vi "Configurator.vi"(8 "error in (no error)":errorcluster) -> (0 "error out":errorcluster)   [LabVIEW 2014]
uses:
  <vilib>/userdefined/High Color/IMAQdx.ctl
  ImageCluster.ctl
  <vilib>/vision/Image Controls.llb/IMAQ Image.ctl
  STD - Tap Mode.ctl
  FlappyHeightPoint.ctl
  <vilib>/LabVIEW Hacker/LINX/Private/Type Defs/User Platform.ctl
  <vilib>/LabVIEW Hacker/LINX/Private/Type Defs/Interface.ctl
  <vilib>/vision/driver/IMAQdx.llb/IMAQdx Acquisition Mode.ctl
  Globals.vi
  <vilib>/vision/driver/NI_Vision_Acquisition_Software.lvlib
  <vilib>/LabVIEW Hacker/LINX/LVH-LINX.lvlib
panel:
  in  "Proceed":bool
  out "Camera connected":bool
  out "Arduino connected":bool
  out "Flappy template loaded":bool
  out "Pipe template loaded":bool
  in  "Serial Port":refnum<visa-resource-name>="N/A"
  in  "IMAQdx Camera Session":T1 caption="Camera to use"
  out "Camera Information Array":T2(array[cluster]) {"BusType" format="%x"; "SerialNumberLow" format="%.0x"; "SerialNumberHigh" format="%.0x"}
  in  "Pipe Corner Template Path":path
  in  "Flappy Template Path":path
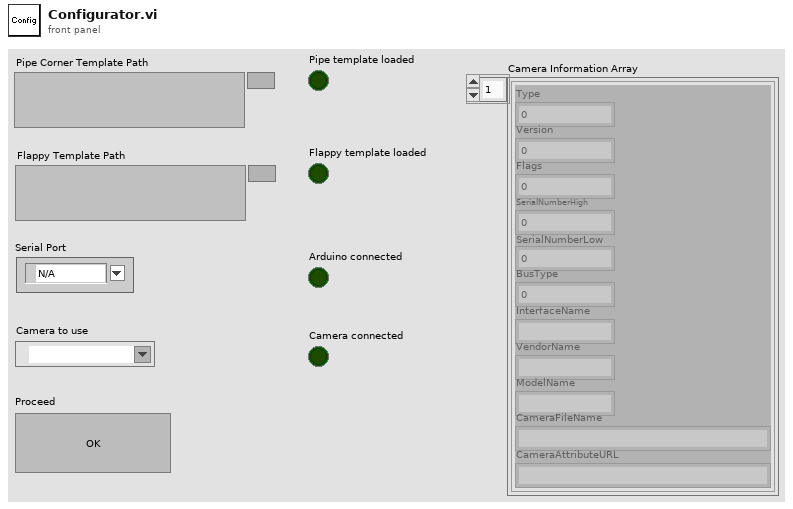
[diagram p1: front panel]
types:
  T1 = typedef "IMAQdx.ctl" = refnum<k21>
  T2 = cluster{"Type":u32, "Version":u32, "Flags":u32, "SerialNumberHigh":u32, "SerialNumberLow":u32, "BusType":u32, "InterfaceName":string, "VendorName":string, "ModelName":string, "CameraFileName":string, "CameraAttributeURL":string}[]
  T3 = typedef "FlappyHeightPoint.ctl" = cluster{"Time (s)":dbl, "Height (px)":dbl}
  T4 = typedef "STD - Tap Mode.ctl" = enum32{"No Action", "Stay Level", "Rise", "Fall", "Calibrate"}
  T5 = typedef "ImageCluster.ctl" = cluster{"Screenshot":T6, "Time (s)":dbl}
  T6 = typedef "IMAQ Image.ctl" = refnum<image>
  T7 = typedef "LVH-LINX.lvlib/Interface.ctl" = enum16{"Serial", "TCP"}
  T8 = typedef "LVH-LINX.lvlib/User Platform.ctl" = enum16{"Default", "LINX", "myRIO"}
  T9 = typedef "NI_Vision_Acquisition_Software.lvlib/IMAQdx Acquisition Mode.ctl" = enum32{"One Shot", "Continuous"}
  T10 = typedef "LVH-LINX.lvlib/LINX Ref.ctl" = cluster{"Platform":T11, "Interface":T7, "LINX Device Config":T12}
  T11 = typedef "LVH-LINX.lvlib/Platform.ctl" = enum16{"LINX", "myRIO"}
  T12 = typedef "LVH-LINX.lvlib/Device.lvlib/LINX Device Config.ctl" = cluster{"Interface":T7, "COM Port":refnum<visa-resource-name>, "TCP Configuration":T13, "Device Family":T14, "Device ID":u8, "Device Name":string, "TCP Ref":refnum<k5>}
  T13 = typedef "LVH-LINX.lvlib/Device.lvlib/TCP Config.ctl" = cluster{"IP Address":string, "Port":u16}
  T14 = typedef "LVH-LINX.lvlib/Device Family.ctl" = enum8{"National Instruments", "Digilent", "Arduino"}
  T15 = typedef "Image Type" = u32
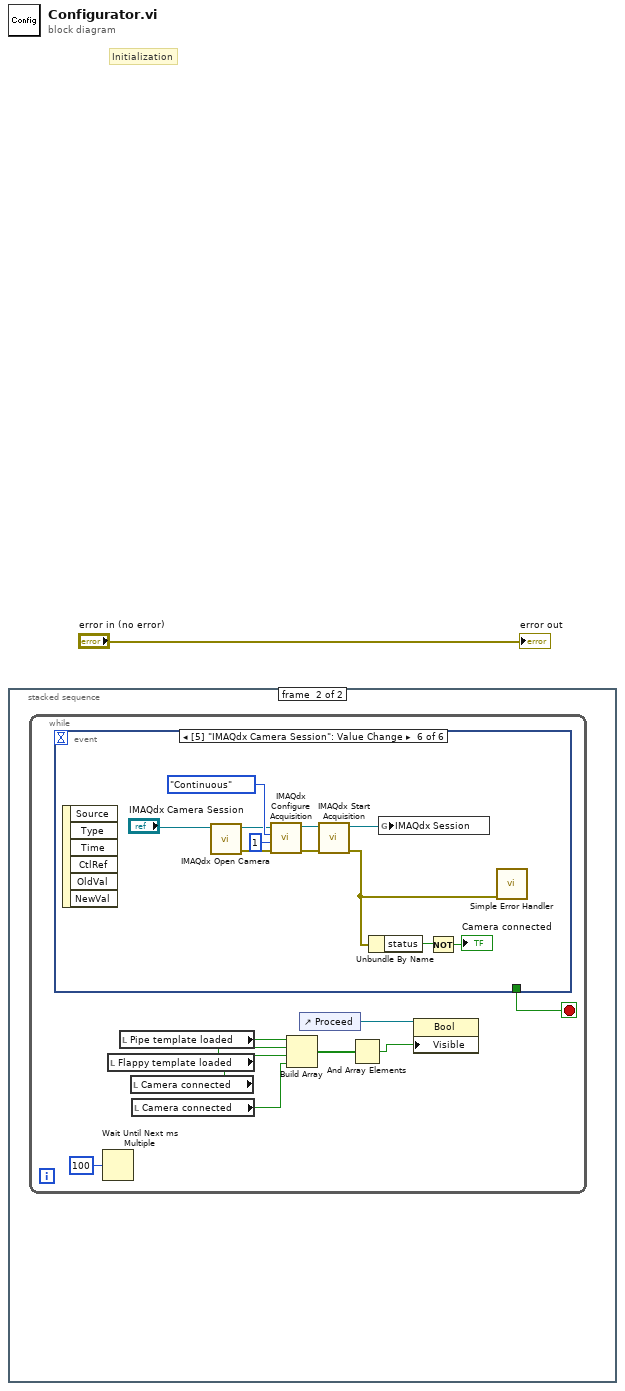
[diagram p0: block diagram]
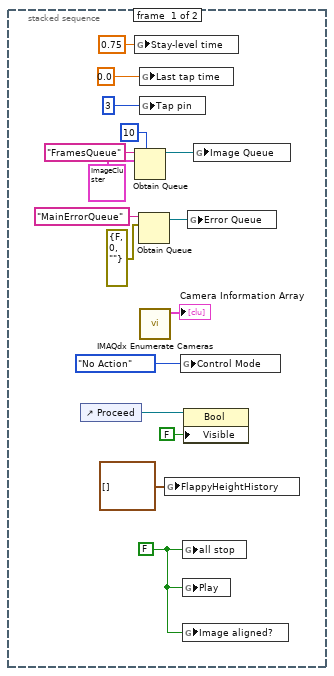
[diagram p2: hidden frame]
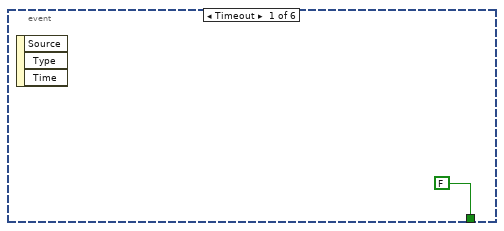
[diagram p3: hidden frame]
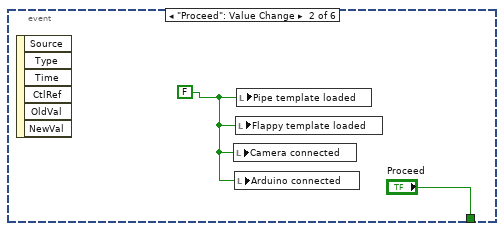
[diagram p4: hidden frame]
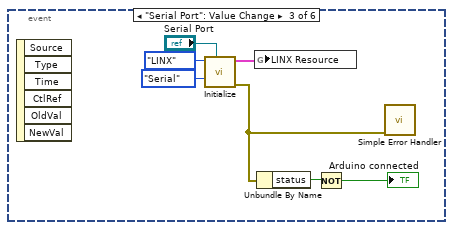
[diagram p5: hidden frame]
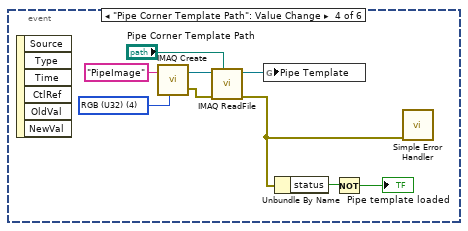
[diagram p6: hidden frame]
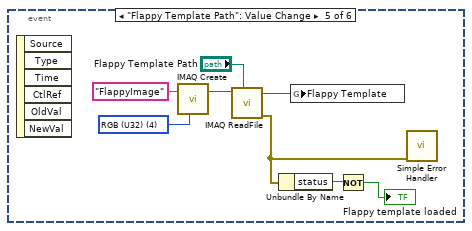
[diagram p7: hidden frame]
diagram:
  # "Initialization"
  n1 = stacked-sequence {
    frame #0 {
      w2 = FALSE ("all stop")
      n2 = control-ref of="Proceed"() -> (w5:refnum<vi>)
      n3 = global write "Globals.vi" "Stay-level time"(0.75 ("Stay-level time")) -> ()
      n4 = Obtain Queue(max queue size (-1, unlimited)=10, name (unnamed)="FramesQueue", element data type=T5 {"Screenshot"=refnum, "Time (s)"=0.0}) -> (queue out=w14:refnum<queue>)  [unwired: 2 in, 2 out]
      n5 = Obtain Queue(name (unnamed)="MainErrorQueue", element data type=errorcluster {"status"=FALSE, "code"=0, "source"=""} ("error constant")) -> (queue out=w8:refnum<queue>)  [unwired: 3 in, 2 out]
      n6 = global write "Globals.vi" "Last tap time"(0.0 ("Last tap time")) -> ()
      n7 = global write "Globals.vi" "Tap pin"(u32 3 ("Tap pin")) -> ()
      n8 = call <vilib>:"IMAQdx Enumerate Cameras.vi"() -> ("Camera Information Array"=→"Camera Information Array":T2)  [unwired: 10 in, 1 out]
      n9 = global write "Globals.vi" "FlappyHeightHistory"(T3[] [] ("FlappyHeightHistory")) -> ()
      n10 = global write "Globals.vi" "Control Mode"(STD_-_Tap_Mode."No Action" ("Control Mode")) -> ()
      n11 = global write "Globals.vi" "all stop"(w2) -> ()
      n12 = global write "Globals.vi" "Play"(w2) -> ()
      n13 = global write "Globals.vi" "Image aligned?"(w2) -> ()
      n14 = property class="Bool"(reference=w5, "Visible"=FALSE) -> ()  [unwired: 1 in, 2 out]
      n15 = global write "Globals.vi" "Error Queue"(w8) -> ()
      n16 = global write "Globals.vi" "Image Queue"(w14) -> ()
    }
    frame #1 {
      n17 = while {
        stop <- w26 stop-if-true
        n18 = event shown="[5] \"IMAQdx Camera Session\": Value Change" {
          selector: _ -> [_ _ _ _ _ _]
          dyn-events: _ -> [_ _ _ _ _ _]
          timeout: _ -> [_ _ _ _ _ _]
          tunnel: [FALSE "Proceed" _ _ _ _] -> w26
          event Timeout {
            n19 = event-data() -> ()  [unwired: 1 in, 3 out]
          }
          event "Proceed": Value Change {
            w28 = FALSE
            n20 = event-data() -> ()  [unwired: 1 in, 6 out]
            n21 = local write "Camera connected"(w28) -> ()
            n22 = local write "Arduino connected"(w28) -> ()
            n23 = local write "Flappy template loaded"(w28) -> ()
            n24 = local write "Pipe template loaded"(w28) -> ()
          }
          event "Serial Port": Value Change {
            n25 = event-data() -> ()  [unwired: 1 in, 6 out]
            n26 = call <vilib>:"Initialize.vi"("Serial Port"="Serial Port", "Interface"=Interface."Serial", "Platform"=User_Platform."LINX") -> ("Error Out"=w30:errorcluster, "LINX Ref"=w36:T10)  [unwired: 6 in, 1 out]
            n27 = global write "Globals.vi" "LINX Resource"(w36) -> ()
            n28 = Unbundle By Name(w30) -> ("status"=w32:bool)
            n29 = Not(x=w32) -> (.not. x?=→"Arduino connected":bool)
            n30 = call <vilib>:"Simple Error Handler.vi"("error in (no error)"=w30) -> ()  [unwired: 4 in, 5 out]
          }
          event "Pipe Corner Template Path": Value Change {
            w44 = T15 4 items=["Grayscale (U8)", "Grayscale (I16)", "Grayscale (SGL)", "Complex (CSG)", "RGB (U32)", "HSL (U32)", "RGB (U64)", "Grayscale (U16)"] ("Image Type")
            n31 = event-data() -> ()  [unwired: 1 in, 6 out]
            n32 = call "IMAQ Create"("Image Name"="PipeImage", "Image Type"=w44) -> ("New Image"=w42:T6, "error out"=w40:errorcluster)  [unwired: 3 in]
            n33 = call "IMAQ ReadFile"("File Path"="Pipe Corner Template Path", "error in (no error)"=w40, "Image"=w42) -> ("error out"=w38:errorcluster, "Image Out"=w45:T6)  [unwired: 4 in, 3 out]
            n34 = global write "Globals.vi" "Pipe Template"(w45) -> ()
            n35 = Unbundle By Name(w38) -> ("status"=w39:bool)
            n36 = Not(x=w39) -> (.not. x?=→"Pipe template loaded":bool)
            n37 = call <vilib>:"Simple Error Handler.vi"("error in (no error)"=w38) -> ()  [unwired: 4 in, 5 out]
          }
          event "Flappy Template Path": Value Change {
            w52 = T15 4 items=["Grayscale (U8)", "Grayscale (I16)", "Grayscale (SGL)", "Complex (CSG)", "RGB (U32)", "HSL (U32)", "RGB (U64)", "Grayscale (U16)"] ("Image Type")
            n38 = event-data() -> ()  [unwired: 1 in, 6 out]
            n39 = call "IMAQ Create"("Image Name"="FlappyImage", "Image Type"=w52) -> ("New Image"=w50:T6)  [unwired: 3 in, 1 out]
            n40 = call "IMAQ ReadFile"("File Path"="Flappy Template Path", "Image"=w50) -> ("error out"=w47:errorcluster, "Image Out"=w53:T6)  [unwired: 5 in, 3 out]
            n41 = Unbundle By Name(w47) -> ("status"=w48:bool)
            n42 = global write "Globals.vi" "Flappy Template"(w53) -> ()
            n43 = Not(x=w48) -> (.not. x?=→"Flappy template loaded":bool)
            n44 = call <vilib>:"Simple Error Handler.vi"("error in (no error)"=w47) -> ()  [unwired: 4 in, 5 out]
          }
          event Value Change {
            n45 = event-data() -> ()  [unwired: 1 in, 6 out]
            n46 = call <vilib>:"IMAQdx Open Camera.vi"("Session In"="IMAQdx Camera Session") -> ("error out"=w57:errorcluster, "Session Out"=w58:T1)  [unwired: 9 in]
            n47 = call <vilib>:"IMAQdx Configure Acquisition.vi"("error in"=w57, "Number of Buffers"=u32 1, "Continuous?"=IMAQdx_Acquisition_Mode."Continuous", "Session In"=w58) -> ("error out"=w61:errorcluster, "Session Out"=w62:T1)  [unwired: 6 in]
            n48 = call <vilib>:"IMAQdx Start Acquisition.vi"("error in"=w61, "Session In"=w62) -> ("error out"=w55:errorcluster, "Session Out"=w64:T1)  [unwired: 8 in]
            n49 = Unbundle By Name(w55) -> ("status"=w56:bool)
            n50 = global write "Globals.vi" "IMAQdx Session"(w64) -> ()
            n51 = Not(x=w56) -> (.not. x?=→"Camera connected":bool)
            n52 = call <vilib>:"Simple Error Handler.vi"("error in (no error)"=w55) -> ()  [unwired: 4 in, 5 out]
          }
        }
        n53 = Wait Until Next ms Multiple(millisecond multiple=u32 100) -> ()  [unwired: 1 out]
        n54 = local read "Flappy template loaded"() -> (w22:bool)
        n55 = local read "Pipe template loaded"() -> (w21:bool)
        n56 = local read "Camera connected"() -> (w19:bool)
        n57 = local read "Camera connected"() -> (w18:bool)
        n58 = Build Array(w21, w22, w19, w18) -> (w20:bool[])
        n59 = control-ref of="Proceed"() -> (w24:refnum<vi>)
        n60 = And Array Elements(Boolean array=w20) -> (logical AND=w23:bool)
        n61 = property class="Bool"(reference=w24, "Visible"=w23) -> ()  [unwired: 1 in, 2 out]
      }
    }
  }
  "error out" <- "error in (no error)"
